vi "Replace Array Variable.vi"(1 "In array":dbl[](array[numeric]), 2 "Cluster Key":u16, 3 "New x Value":dbl) -> (0 "Out Array":dbl[](array[numeric]))   [LabVIEW 2020]
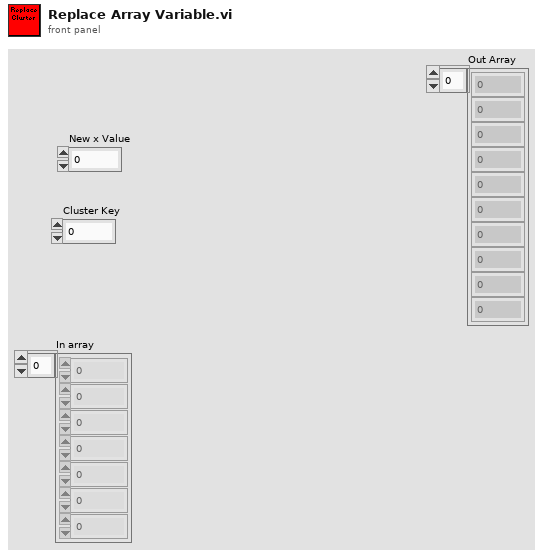
[diagram p1: front panel]
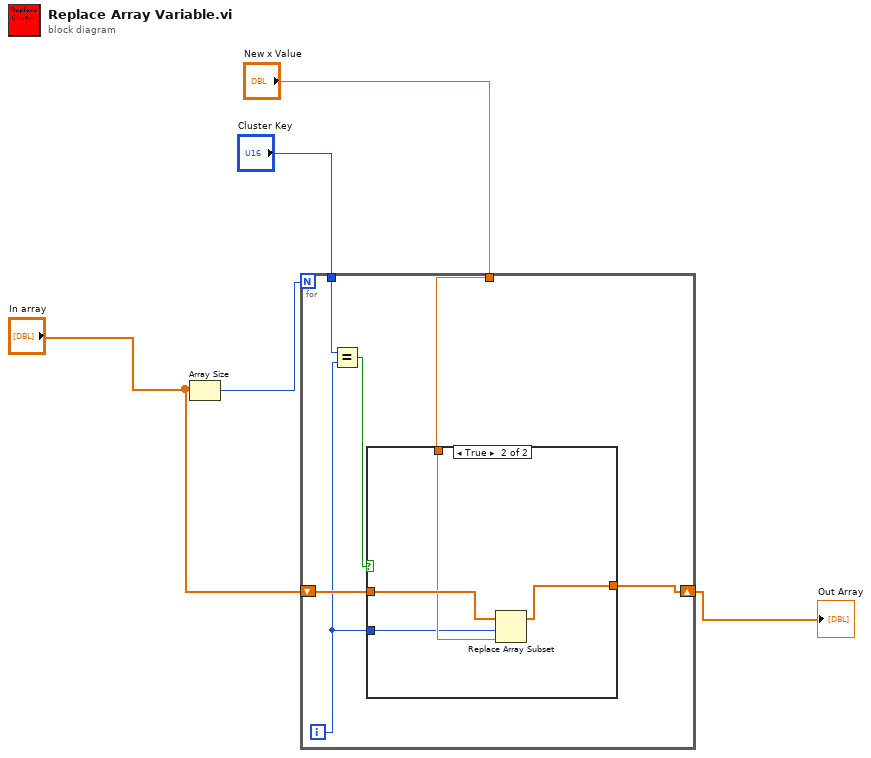
[diagram p0: block diagram]
diagram:
  n1 = Array Size(array="In array") -> (size(s)=w4:i32)
  n2 = for {
    N: w4 -> [_]
    shift-right: [w11] -> w5
    shift-left: "In array" -> [w10]
    tunnel: "Cluster Key" -> [w9]
    tunnel: "New x Value" -> [w7]
    i -> [w6]
    n3 = Equal?(x=w9, y=w6) -> (x = y?=w8:bool)
    n4 = case shown="True" w8 {
      tunnel: [w12 w13] -> w11
      tunnel: w10 -> [w12 w16]
      tunnel: w7 -> [_ w15]
      tunnel: w6 -> [_ w14]
      frame False {
      }
      frame True {
        n5 = Replace Array Subset(array=w16, new element=w15, index=w14) -> (w13:dbl[])
      }
    }
  }
  "Out Array" <- w5
